vi "Launcher General.vi"() -> ()   [LabVIEW 2019]
uses:
  <vilib>/ActorFramework/Message Enqueuer/Message Enqueuer.lvclass
  <vilib>/ActorFramework/Message Enqueuer/Message Enqueuer.lvclass/Message Enqueuer.ctl
  GUI_Actor/GUI_Actor.lvclass
  C:/Program Files/National Instruments/LabVIEW 2019/vi.lib/ActorFramework/Actor/Actor.lvclass
  Contador_Bin_Actor/Contador_Bin_Actor.lvclass
  <vilib>/ActorFramework/Message Enqueuer/Enqueue.vi
  <vilib>/ActorFramework/Stop Msg/Stop Msg.lvclass
  C:/Program Files/National Instruments/LabVIEW 2019/vi.lib/ActorFramework/Message/Message.lvclass
  <vilib>/ActorFramework/Message Priority Queue/Priority Enqueue.vi
  <vilib>/ActorFramework/Actor/Actor.lvclass
panel:
  in  "Visualizar Generador de Funciones":u16(ring)
  in  "Close CB":bool
  in  "Add CB":bool
  in  "Visualizar Contador Binario":u16(ring)
  in  "Close GF":bool
  in  "Add GF":bool
  in  "stop":bool
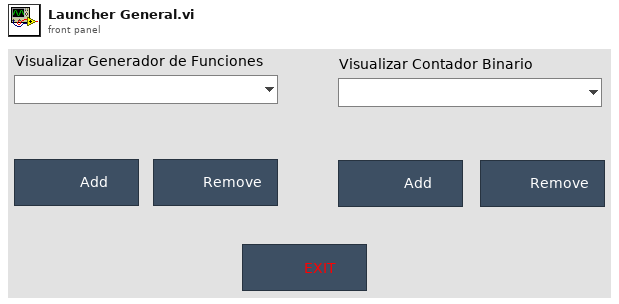
[diagram p1: front panel]
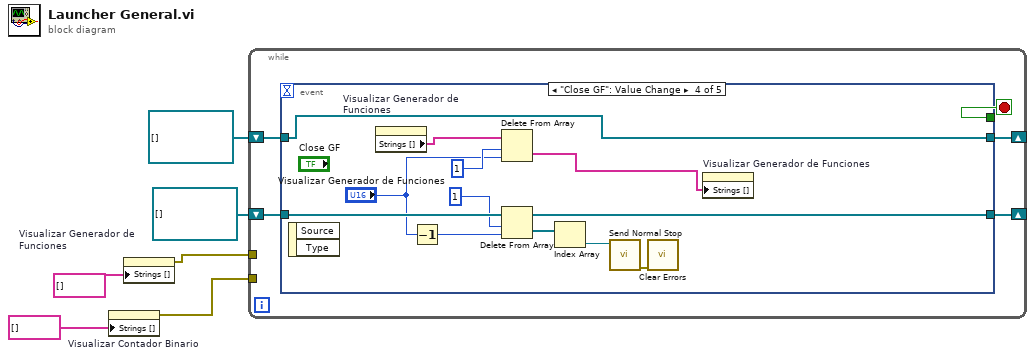
[diagram p0: block diagram]
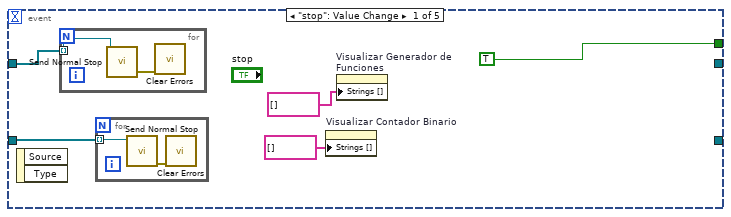
[diagram p2: hidden frame]
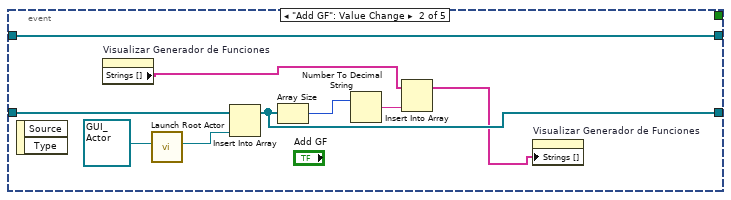
[diagram p3: hidden frame]
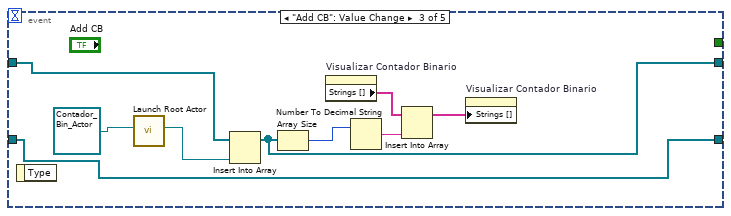
[diagram p4: hidden frame]
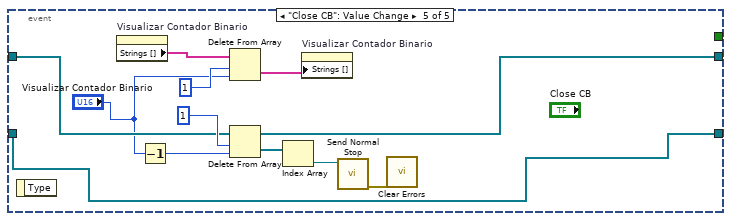
[diagram p5: hidden frame]
diagram:
  n1 = property on="Visualizar Contador Binario" class="Ring (strict)"("Strings []"=string[] []) -> (error out=w1:errorcluster)  [unwired: 2 in, 1 out]
  n2 = property on="Visualizar Generador de Funciones" class="Ring (strict)"("Strings []"=string[] [] ("Item Names")) -> (error out=w2:errorcluster)  [unwired: 2 in, 1 out]
  n3 = while {
    shift-right: [w9] -> _
    shift-left: refnum<class "Message Enqueuer.lvclass">[] [] ("Actor's Enqueuer") -> [w10]
    shift-right: [w7] -> _
    shift-left: refnum<class "Message Enqueuer.lvclass">[] [] ("Actor's Enqueuer") -> [w8]
    tunnel: w2 -> [_]
    tunnel: w1 -> [_]
    stop <- w11 stop-if-true
    n4 = event shown="[3] \"Close GF\": Value Change" {
      selector: _ -> [_ _ _ _ _]
      dyn-events: _ -> [_ _ _ _ _]
      timeout: _ -> [_ _ _ _ _]
      tunnel: [TRUE ("stop") _ _ _ _] -> w11
      tunnel: w10 -> [w14 w27 w30 w50 w55]
      tunnel: [_ w26 w30 w48 w55] -> w9
      tunnel: w8 -> [w15 w23 w32 w43 w57]
      tunnel: [_ w23 w31 w43 w56] -> w7
      event "stop": Value Change {
        n5 = event-data() -> ()  [unwired: 1 in, 2 out]
        n6 = for {
          tunnel: w15 -> [w20] mode=indexing
          n7 = call <vilib>:"Send Normal Stop.vi"("Message Enqueuer"=w20) -> ("error out"=w19:errorcluster)  [unwired: 10 in]
          n8 = call <vilib>:"Clear Errors.vi"("error in (no error)"=w19) -> ()  [unwired: 5 in, 2 out]
        }
        n9 = for {
          tunnel: w14 -> [w18] mode=indexing
          n10 = call <vilib>:"Send Normal Stop.vi"("Message Enqueuer"=w18) -> ("error out"=w17:errorcluster)  [unwired: 10 in]
          n11 = call <vilib>:"Clear Errors.vi"("error in (no error)"=w17) -> ()  [unwired: 5 in, 2 out]
        }
        n12 = property on="Visualizar Contador Binario" class="Ring (strict)"("Strings []"=string[] []) -> ()  [unwired: 2 in, 2 out]
        n13 = property on="Visualizar Generador de Funciones" class="Ring (strict)"("Strings []"=string[] []) -> ()  [unwired: 2 in, 2 out]
      }
      event "Add GF": Value Change {
        n14 = event-data() -> ()  [unwired: 1 in, 2 out]
        n15 = property on="Visualizar Generador de Funciones" class="Ring (strict)"() -> ("Strings []"=w22:string[])  [unwired: 2 in, 2 out]
        n16 = call <vilib>:"Launch Root Actor.vi"("Actor"=refnum<class "GUI_Actor.lvclass"> refnum ("GUI_Actor.lvlib:GUI_Actor.lvclass")) -> ("Actor's Enqueuer"=w28:refnum<class "Message Enqueuer.lvclass">)  [unwired: 9 in, 1 out]
        n17 = Insert Into Array(array=w27, new element=w28) -> (w26:refnum<class "Message Enqueuer.lvclass">[])  [unwired: 1 in]
        n18 = Array Size(array=w26) -> (size(s)=w25:i32)
        n19 = Number To Decimal String(number=w25) -> (decimal integer string=w24:string)  [unwired: 1 in]
        n20 = Insert Into Array(array=w22, new element=w24) -> (w21:string[])  [unwired: 1 in]
        n21 = property on="Visualizar Generador de Funciones" class="Ring (strict)"("Strings []"=w21) -> ()  [unwired: 2 in, 2 out]
      }
      event "Add CB": Value Change {
        n22 = event-data() -> ()  [unwired: 1 in, 1 out]
        n23 = call <vilib>:"Launch Root Actor.vi"("Actor"=refnum<class "Contador_Bin_Actor.lvclass"> refnum ("Contador_Bin_Actor.lvlib:Contador_Bin_Actor.lvclass")) -> ("Actor's Enqueuer"=w38:refnum<class "Message Enqueuer.lvclass">)  [unwired: 9 in, 1 out]
        n24 = Insert Into Array(array=w32, new element=w38) -> (w31:refnum<class "Message Enqueuer.lvclass">[])  [unwired: 1 in]
        n25 = Array Size(array=w31) -> (size(s)=w37:i32)
        n26 = property on="Visualizar Contador Binario" class="Ring (strict)"() -> ("Strings []"=w33:string[])  [unwired: 2 in, 2 out]
        n27 = Number To Decimal String(number=w37) -> (decimal integer string=w36:string)  [unwired: 1 in]
        n28 = Insert Into Array(array=w33, new element=w36) -> (w34:string[])  [unwired: 1 in]
        n29 = property on="Visualizar Contador Binario" class="Ring (strict)"("Strings []"=w34) -> ()  [unwired: 2 in, 2 out]
      }
      event "Close GF": Value Change {
        n30 = event-data() -> ()  [unwired: 1 in, 2 out]
        n31 = property on="Visualizar Generador de Funciones" class="Ring (strict)"() -> ("Strings []"=w41:string[])  [unwired: 2 in, 2 out]
        n32 = Decrement(x="Visualizar Generador de Funciones") -> (x-1=w44:u16)
        n33 = Delete From Array(array=w41, length=1, index="Visualizar Generador de Funciones") -> (deleted portion=w42:string[])  [unwired: 1 out]
        n34 = Delete From Array(array=w50, length=1, index=w44) -> (deleted portion=w47:refnum<class "Message Enqueuer.lvclass">[], array with subset deleted=w48:refnum<class "Message Enqueuer.lvclass">[])
        n35 = Index Array(array=w47) -> (element=w46:refnum<class "Message Enqueuer.lvclass">)  [unwired: 1 in]
        n36 = call <vilib>:"Send Normal Stop.vi"("Message Enqueuer"=w46) -> ("error out"=w39:errorcluster)  [unwired: 10 in]
        n37 = call <vilib>:"Clear Errors.vi"("error in (no error)"=w39) -> ()  [unwired: 5 in, 2 out]
        n38 = property on="Visualizar Generador de Funciones" class="Ring (strict)"("Strings []"=w42) -> ()  [unwired: 2 in, 2 out]
      }
      event "Close CB": Value Change {
        n39 = event-data() -> ()  [unwired: 1 in, 1 out]
        n40 = property on="Visualizar Contador Binario" class="Ring (strict)"() -> ("Strings []"=w53:string[])  [unwired: 2 in, 2 out]
        n41 = Decrement(x="Visualizar Contador Binario") -> (x-1=w58:u16)
        n42 = Delete From Array(array=w53, length=1, index="Visualizar Contador Binario") -> (deleted portion=w54:string[])  [unwired: 1 out]
        n43 = Delete From Array(array=w57, length=1, index=w58) -> (deleted portion=w61:refnum<class "Message Enqueuer.lvclass">[], array with subset deleted=w56:refnum<class "Message Enqueuer.lvclass">[])
        n44 = Index Array(array=w61) -> (element=w60:refnum<class "Message Enqueuer.lvclass">)  [unwired: 1 in]
        n45 = property on="Visualizar Contador Binario" class="Ring (strict)"("Strings []"=w54) -> ()  [unwired: 2 in, 2 out]
        n46 = call <vilib>:"Send Normal Stop.vi"("Message Enqueuer"=w60) -> ("error out"=w51:errorcluster)  [unwired: 10 in]
        n47 = call <vilib>:"Clear Errors.vi"("error in (no error)"=w51) -> ()  [unwired: 5 in, 2 out]
      }
    }
  }
